vi "Wait Untill All Done.vi"(8 "error in (no error)":errorcluster, 11 "HSDIO Sessions In":refnum<k15>[](array[refnum])) -> (0 "error out":errorcluster, 3 "HSDIO Sessions Out":refnum<k15>[](array[refnum]))   [LabVIEW 2013]
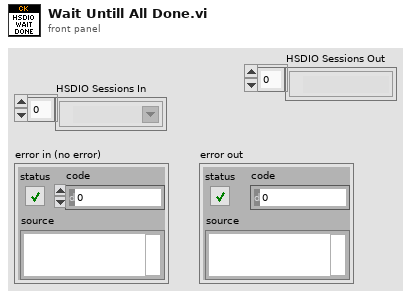
[diagram p1: front panel]
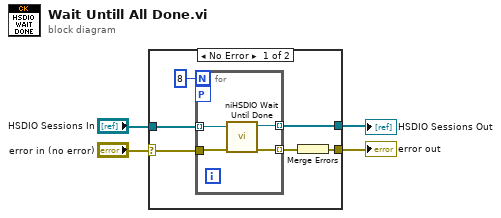
[diagram p0: block diagram]
diagram:
  n1 = case shown="No Error" "error in (no error)" {
    selector: "error in (no error)" -> [w5 w16]
    tunnel: "HSDIO Sessions In" -> [w9 w15]
    tunnel: [w8 w16] -> w3
    tunnel: [w6 w15] -> w2
    frame No Error {
      n2 = for {
        N: 8 -> [_]
        tunnel: w5 -> [w14]
        tunnel: [w13] -> w7 mode=indexing
        tunnel: w9 -> [w12] mode=indexing
        workers-P: _ -> [_]
        tunnel: [w11] -> w6 mode=indexing
        n3 = call <instrlib>:"niHSDIO Wait Until Done.vi"("error in (no error)"=w14, "instrument handle"=w12) -> ("error out"=w13:errorcluster, "instrument handle out"=w11:refnum<k15>)  [unwired: 8 in]
      }
      n4 = Merge Errors(w7) -> (w8:errorcluster)
    }
    frame Error {
    }
  }
  "error out" <- w3
  "HSDIO Sessions Out" <- w2
